vi "Position Waypoint Number String.vi"(8 "error in (no error)":errorcluster, 10 "Tab Ctrl Ref":refnum<vi>, 11 "Str Refnum":refnum<vi>) -> (0 "error out":errorcluster)   [LabVIEW 2014]
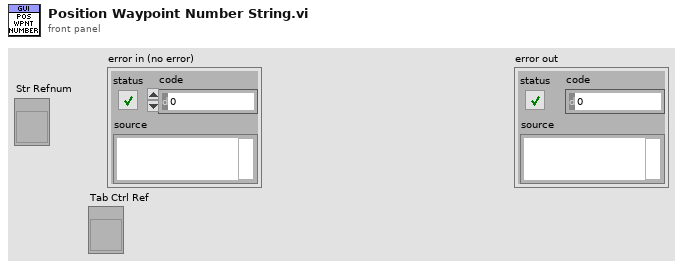
[diagram p1: front panel]
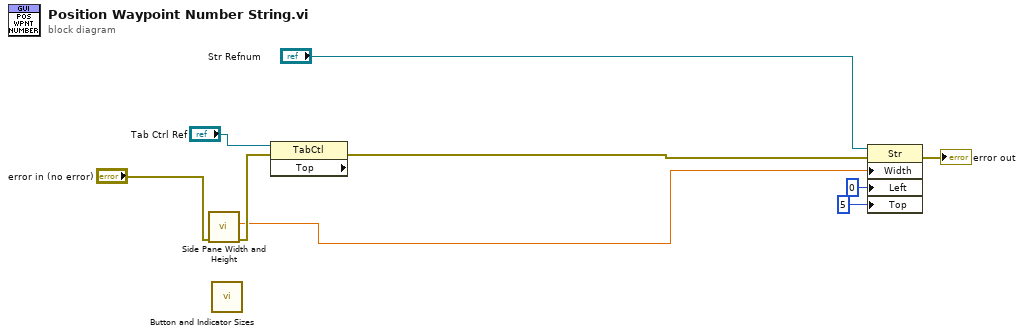
[diagram p0: block diagram]
diagram:
  n1 = call "Side Pane Width and Height.vi"("error in (no error)"="error in (no error)") -> ("error out"=w6:errorcluster, "Width"=w2:dbl)  [unwired: 8 in, 1 out]
  n2 = call "Button and Indicator Sizes.vi"() -> ()  [unwired: 11 in, 5 out]
  n3 = property class="TabCtl" props=["Top"](reference="Tab Ctrl Ref", error in=w6) -> (error out=w1:errorcluster)  [unwired: 2 out]
  n4 = property class="Str"(reference="Str Refnum", error in=w1, "Width"=w2, "Left"=0 ("Position:Left"), "Top"=5 ("Position:Top")) -> (error out=→"error out":errorcluster)  [unwired: 1 out]
